vi "OAT Remove Boundaries.vi"(4 "indices to remove":i32[](array[numeric]), 6 "array 2 in":i32[](array[numeric]), 7 "array 1 in":i32[](array[numeric])) -> (2 "array 2 out":i32[](array[numeric]), 3 "array 1 out":i32[](array[numeric]))   [LabVIEW 2017, in "SoundVib_Gabor.lvlib"]
uses:
  <vilib>/addons/Sound and Vibration/Order Analysis/Gabor Order Tracking/SoundVib_Gabor.lvlib
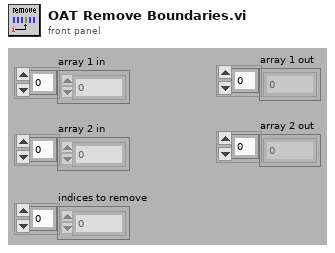
[diagram p1: front panel]
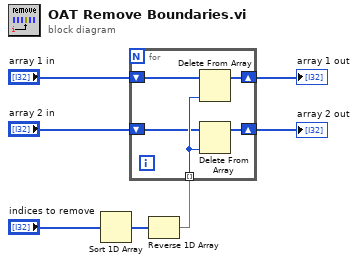
[diagram p0: block diagram]
diagram:
  n1 = Sort 1D Array(array="indices to remove") -> (sorted array=w3:i32[])
  n2 = Reverse 1D Array(array=w3) -> (reversed array=w1:i32[])
  n3 = for {
    tunnel: w1 -> [w12] mode=indexing
    shift-right: [w10] -> w6
    shift-left: "array 1 in" -> [w11]
    shift-right: [w8] -> w7
    shift-left: "array 2 in" -> [w9]
    n4 = Delete From Array(array=w11, index=w12) -> (array with subset deleted=w10:i32[])  [unwired: 1 in, 1 out]
    n5 = Delete From Array(array=w9, index=w12) -> (array with subset deleted=w8:i32[])  [unwired: 1 in, 1 out]
  }
  "array 2 out" <- w7
  "array 1 out" <- w6
